vi "DMC CLI Caraya Command Line Example.vi"() -> ()   [LabVIEW 2023]
panel:
  in  "Report Name":string="Caraya Test Results"
  out "standard error":string
  in  "Working Directory":path=path ""
  out "error out":errorcluster
  out "return code":i32
  out "standard output":string
  in  "Run Caraya?":bool
  out "CMD String":string
  in  "Verbose?":bool=TRUE
  in  "Excluded Bookmarks":string[](array[string])
  in  "Included Bookmarks":string[](array[string])
  in  "Report Directory":path
  in  "Source":path
  in  "LabVIEW Year":string="2023"
  in  "Timeout (ms)":i32=240000
  # "g-cli (optional)--lv-ver [LV_Year] (optional)--timeout [ms Timeout] \"DMC CLI Caraya\" -- [arguments]\n\n-------optional arguments-------\n-source <relative to working directory paths, comma delimited. Defaults to working directory> (Can be .vi, folders, .lvproj)\n-reportdir <absolute or relative to working directory relative path to report output directory. Defaults to workingdir/Reports>\n-reportname <string name of xml report. Defaults to Caraya Test Results.xml>\n-include <comma seperated string of all Bookmarks Unit Tests must have to be included. Defaults to include all>\n-exclude <comma seperated string of all Bookmarks Unit Tests cannot have, or will be excluded. Defaults to none>\n-vurbose <Flag to set report verbose>\n-help <Returns this help information>"
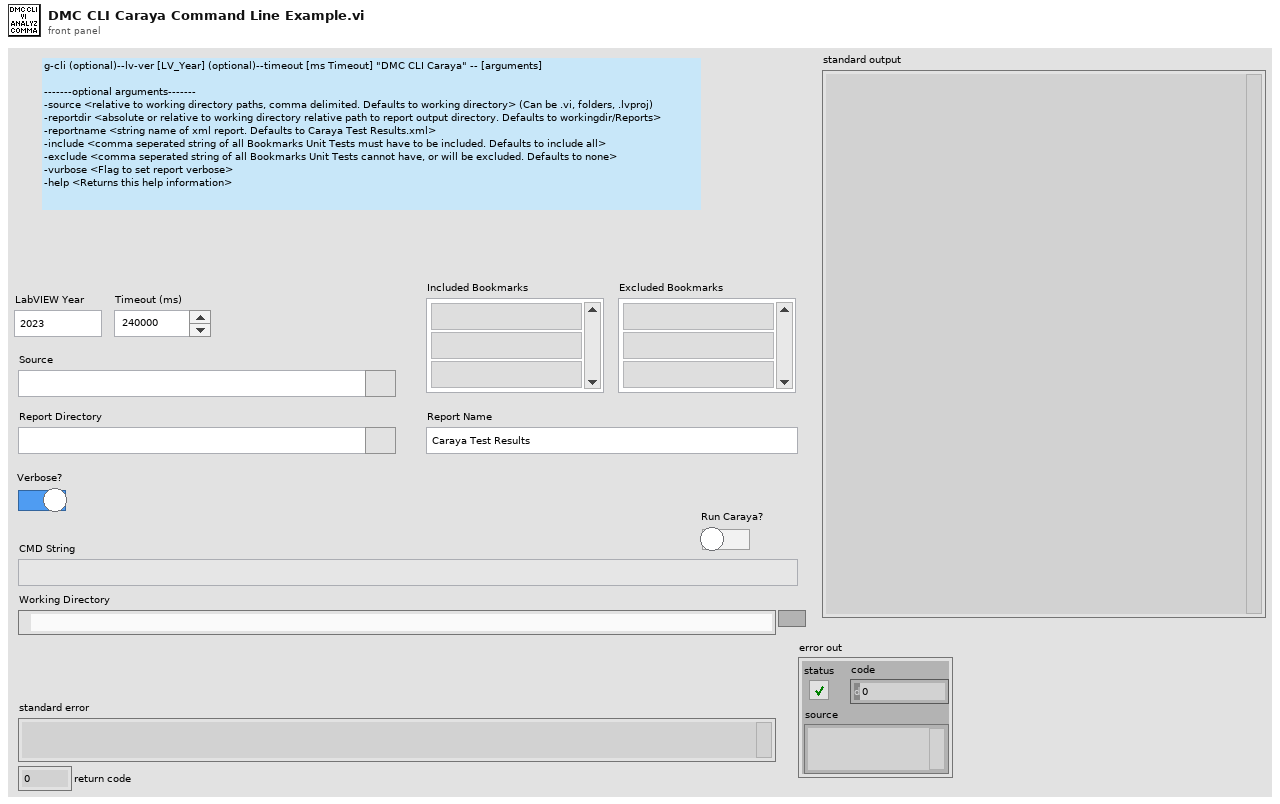
[diagram p1: front panel]
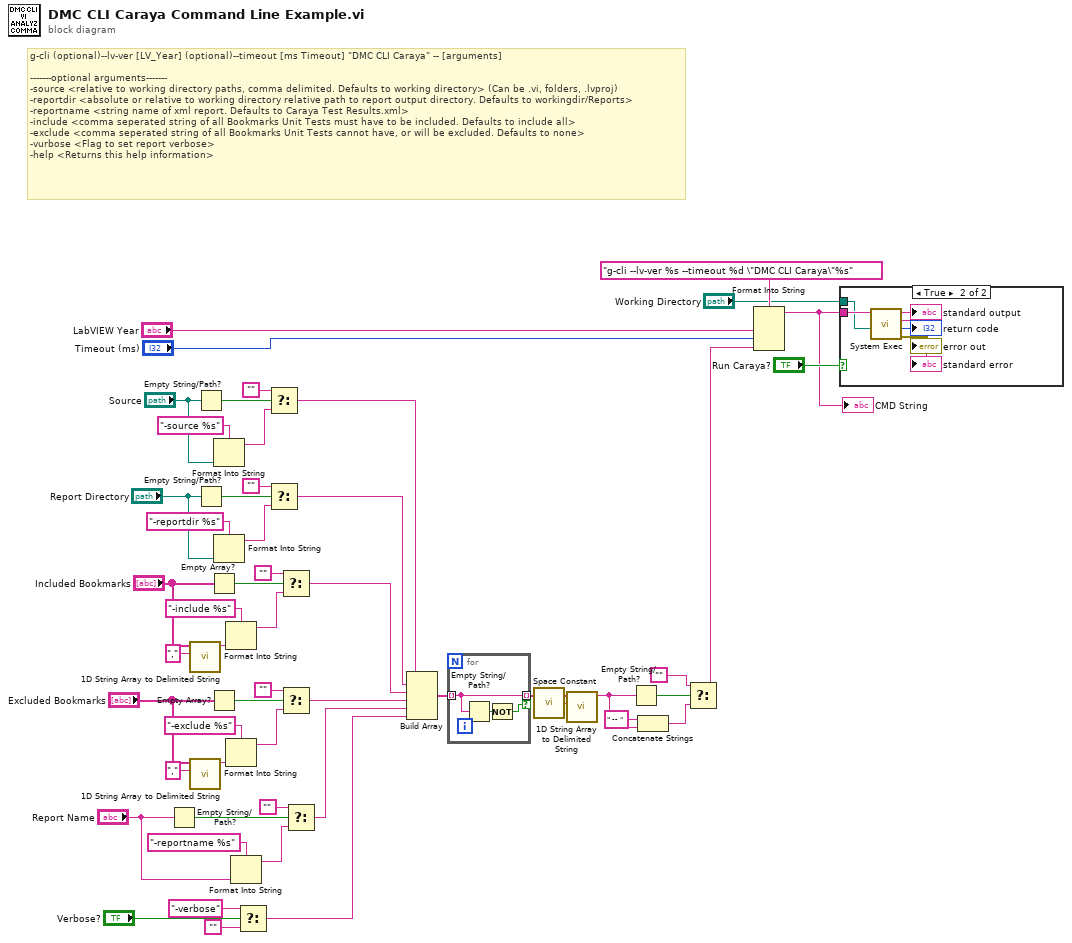
[diagram p0: block diagram]
diagram:
  # "g-cli (optional)--lv-ver [LV_Year] (optional)--timeout [ms Timeout] \"DMC CLI Caraya\" -- [arguments]\n\n-------optional arguments-------\n-source <relative to working directory paths, comma delimited. Defaults to working directory> (Can be .vi, folders, .lvproj)\n-reportdir <absolute or relative to working directory relative path to report output directory. Defaults to workingdir/Reports>\n-reportname <string name of xml report. Defaults to Caraya Test Results.xml>\n-include <comma seperated string of all Bookmarks Unit Tests must have to be included. Defaults to include all>\n-exclude <comma seperated string of all Bookmarks Unit Tests cannot have, or will be excluded. Defaults to none>\n-vurbose <Flag to set report verbose>\n-help <Returns this help information>"
  n1 = Empty String/Path?(string/path="Report Name") -> (empty?=w1:bool)
  n2 = call <vilib>:"1D String Array to Delimited String.vi"("delimiter"=",", "string array"="Included Bookmarks") -> ("delimited string"=w35:string)  [unwired: 9 in]
  n3 = call <vilib>:"1D String Array to Delimited String.vi"("delimiter"=",", "string array"="Excluded Bookmarks") -> ("delimited string"=w32:string)  [unwired: 9 in]
  n4 = Empty String/Path?(string/path="Source") -> (empty?=w50:bool)
  n5 = Empty String/Path?(string/path="Report Directory") -> (empty?=w42:bool)
  n6 = Empty Array?(array="Included Bookmarks") -> (empty?=w34:bool)
  n7 = Empty Array?(array="Excluded Bookmarks") -> (empty?=w33:bool)
  n8 = Format Into String(format string="-source %s", "Source") -> (resulting string=w46:string)  [unwired: 2 in, 1 out]
  n9 = Format Into String(format string="-reportdir %s", "Report Directory") -> (resulting string=w45:string)  [unwired: 2 in, 1 out]
  n10 = Format Into String(format string="-include %s", w35) -> (resulting string=w40:string)  [unwired: 2 in, 1 out]
  n11 = Format Into String(format string="-exclude %s", w32) -> (resulting string=w28:string)  [unwired: 2 in, 1 out]
  n12 = Format Into String(format string="-reportname %s", "Report Name") -> (resulting string=w24:string)  [unwired: 2 in, 1 out]
  n13 = Select(t="-verbose", s="Verbose?", f="") -> (s? t:f=w15:string)
  n14 = Select(t="", s=w50, f=w46) -> (s? t:f=w20:string)
  n15 = Select(t="", s=w42, f=w45) -> (s? t:f=w19:string)
  n16 = Select(t="", s=w34, f=w40) -> (s? t:f=w18:string)
  n17 = Select(t="", s=w33, f=w28) -> (s? t:f=w17:string)
  n18 = Select(t="", s=w1, f=w24) -> (s? t:f=w16:string)
  n19 = Build Array(w20, w19, w18, w17, w16, w15) -> (w5:string[])
  n20 = for {
    tunnel: w5 -> [w56] mode=indexing
    tunnel: [w56] -> w4 mode=indexing if=w54
    n21 = Empty String/Path?(string/path=w56) -> (empty?=w55:bool)
    n22 = Not(x=w55) -> (.not. x?=w54:bool)
  }
  n23 = call <vilib>:"Space Constant.vi"() -> ("String"=w14:string)
  n24 = call <vilib>:"1D String Array to Delimited String.vi"("delimiter"=w14, "string array"=w4) -> ("delimited string"=w13:string)  [unwired: 9 in]
  n25 = Empty String/Path?(string/path=w13) -> (empty?=w11:bool)
  n26 = Concatenate Strings(" -- " ("string"), w13) -> (w9:string)
  n27 = Select(t="", s=w11, f=w9) -> (s? t:f=w8:string)
  n28 = Format Into String(format string="g-cli --lv-ver %s --timeout %d \"DMC CLI Caraya\"%s", "LabVIEW Year", "Timeout (ms)", w8) -> (resulting string=w6:string)  [unwired: 2 in, 1 out]
  "CMD String" <- w6
  n29 = case shown="True" "Run Caraya?" {
    tunnel: w6 -> [_ w62]
    tunnel: "Working Directory" -> [_ w58]
    frame False {
    }
    frame True {
      n30 = call <vilib>:"System Exec.vi"("working directory"=w58, "command line"=w62) -> ("error out"=→"error out":errorcluster, "return code"=→"return code":i32, "standard error"=→"standard error":string, "standard output"=→"standard output":string)  [unwired: 6 in]
    }
  }
